vi "Destroy Promise.vi"(8 "error in (no error)":errorcluster, 9 "force destroy? (F)":bool, 11 "Promise in":refnum<class "Promise.lvclass">) -> (0 "error out":errorcluster)   [LabVIEW 2017, in "Promise Future.lvlib" / "Promise.lvclass"]
uses:
  Promise.lvclass
  Promise.lvclass/Promise.ctl
  Future/Future.lvclass
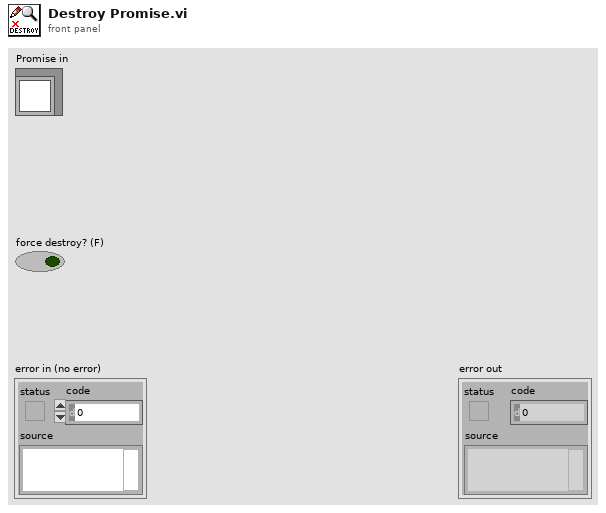
[diagram p1: front panel]
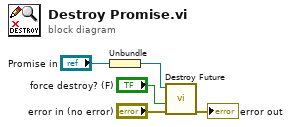
[diagram p0: block diagram]
diagram:
  n1 = Unbundle("Promise in") -> (w2:refnum<class "Future.lvclass">)
  n2 = call "Destroy Future.vi"("error in (no error)"="error in (no error)", "force destroy? (F)"="force destroy? (F)", "Future in"=w2) -> ("error out"=→"error out":errorcluster)  [unwired: 8 in]
